vi "Memory.Pointer.Swap.vi"(8 "error in (no error)":errorcluster, 10 "Pointer B":refnum<class "Memory.Pointer.Void.lvclass">, 11 "Pointer A":refnum<class "Memory.Pointer.Void.lvclass">) -> (0 "error out":errorcluster, 2 "Pointer B'":refnum<class "Memory.Pointer.Void.lvclass">, 3 "Pointer A'":refnum<class "Memory.Pointer.Void.lvclass">)   [LabVIEW 2016, in "LabVIEW Memory Manager.lvlib" / "Memory.Pointer.Void.lvclass"]
uses:
  Memory.Pointer.Void.lvclass
  Memory.Pointer.Void.lvclass/Memory.Pointer.Void.ctl
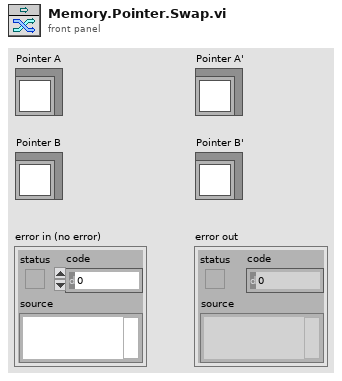
[diagram p1: front panel]
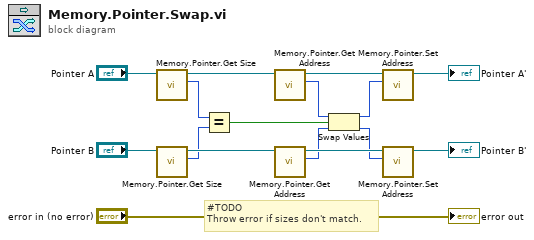
[diagram p0: block diagram]
diagram:
  # "#TODO\nThrow error if sizes don't match."
  n1 = call "Memory.Pointer.Get Size.vi"("Pointer in"="Pointer A") -> ("size"=w14:u64, "Pointer out"=w13:refnum<class "Memory.Pointer.Void.lvclass">)  [unwired: 8 in, 1 out]
  n2 = call "Memory.Pointer.Get Size.vi"("Pointer in"="Pointer B") -> ("size"=w11:u64, "Pointer out"=w12:refnum<class "Memory.Pointer.Void.lvclass">)  [unwired: 8 in, 1 out]
  n3 = Equal?(x=w14, y=w11) -> (x = y?=w2:bool)
  n4 = call "Memory.Pointer.Get Address.vi"("Pointer in"=w13) -> ("address"=w6:u64, "Pointer out"=w8:refnum<class "Memory.Pointer.Void.lvclass">)  [unwired: 8 in, 1 out]
  n5 = call "Memory.Pointer.Get Address.vi"("Pointer in"=w12) -> ("address"=w5:u64, "Pointer out"=w7:refnum<class "Memory.Pointer.Void.lvclass">)  [unwired: 8 in, 1 out]
  n6 = Swap Values(12:w6, 13:w2, 14:w5) -> (1:w4:u64, 3:w3:u64)
  n7 = call "Memory.Pointer.Set Address.vi"("address"=w4, "Pointer in"=w8) -> ("Pointer out"=→"Pointer A'":refnum<class "Memory.Pointer.Void.lvclass">)  [unwired: 8 in, 1 out]
  n8 = call "Memory.Pointer.Set Address.vi"("address"=w3, "Pointer in"=w7) -> ("Pointer out"=→"Pointer B'":refnum<class "Memory.Pointer.Void.lvclass">)  [unwired: 8 in, 1 out]
  "error out" <- "error in (no error)"
